vi "Append Numeric Table to Report.vi"(0 "report in":refnum<class "NI_Standard Report.lvclass">, 1 "column width (1)":dbl=1.0 format="%.2f", 2 "measurement system":u16(ring)=2 caption="measurement system for column width (Default)" items=["US", "Metric", "Default"], 3 "MS Office parameters":T2, 5 "column headers":string[](array[string]), 7 "row headers":string[](array[string]), 9 "numerical data":dbl[][](array[numeric]) format="%.2f", 11 "error in (no error)":errorcluster, 12 "format string (%.3f)":string="%.3f", 13 "separate page?":bool, 14 "show grid lines":bool=TRUE) -> (4 "report out":refnum<class "NI_Standard Report.lvclass">, 8 "range (wd) - start (xl)":T1, 10 "end (xl)":cluster{"row (xl) ":i32, "col (xl) ":i32}, 15 "error out":errorcluster)   [LabVIEW 2017, in "NI_Standard Report.lvclass"]
doc: "Appends a 2D array to a report as a table with the given column width. You can use this polymorphic VI to append an array of strings or numbers. The data type you wire to the <B>text data</B> input determines the polymorphic instance to use."
uses:
  <vilib>/Utility/NIReport.llb/Standard Report/NI_Standard Report.lvclass
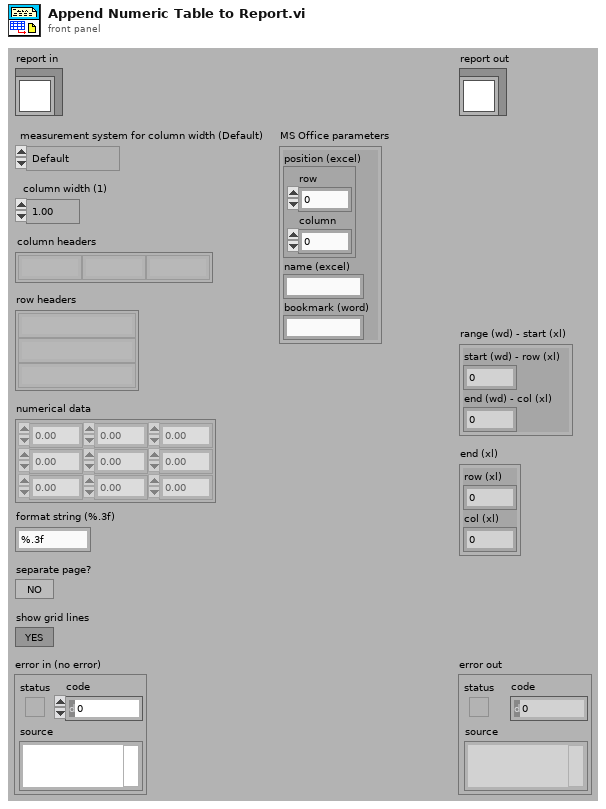
[diagram p1: front panel]
types:
  T1 = cluster{"start (wd) - row (xl) ":i32, "end (wd) - col (xl) ":i32}
  T2 = cluster{"position (excel)":cluster{"row":i32, "column":i32}, "name (excel)":string, "bookmark (word)":string}
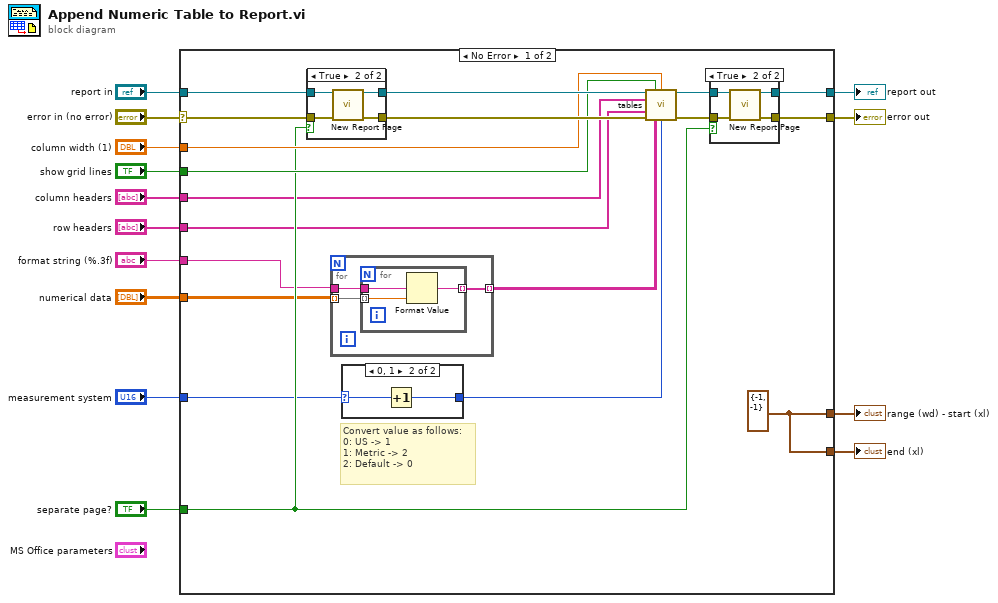
[diagram p0: block diagram]
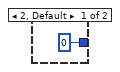
[diagram p2: hidden frame]
diagram:
  n1 = case shown="No Error" "error in (no error)" {
    selector: "error in (no error)" -> [w25 w56]
    tunnel: [w24 w56] -> w13
    tunnel: [w26 w55] -> w11
    tunnel: "report in" -> [w29 w55]
    tunnel: "show grid lines" -> [w22 _]
    tunnel: "format string (%.3f)" -> [w17 _]
    tunnel: "row headers" -> [w19 _]
    tunnel: "column headers" -> [w20 _]
    tunnel: "numerical data" -> [w18 _]
    tunnel: "column width (1)" -> [w23 _]
    tunnel: "separate page?" -> [w21 _]
    tunnel: "measurement system" -> [w16 _]
    tunnel: [w15 _] -> w2
    tunnel: [w15 _] -> w1
    frame No Error {
      w15 = cluster{"row (xl)":i32, "col (xl)":i32} {"row (xl)"=-1, "col (xl)"=-1} ("end (xl)")
      # "Convert value as follows:\n0: US -> 1\n1: Metric -> 2\n2: Default -> 0"
      n2 = case shown="True" w21 {
        tunnel: w29 -> [w50 w54]
        tunnel: w25 -> [w49 w53]
        tunnel: [w50 w52] -> w28
        tunnel: [w49 w51] -> w30
        frame False {
        }
        frame True {
          n3 = call-dynamic "New Report Page.vi"("report in"=w54, "error in (no error)"=w53) -> ("report out"=w52:refnum<class "NI_Standard Report.lvclass">, "error out"=w51:errorcluster)  [unwired: 1 in, 11 out]
        }
      }
      n4 = for {
        tunnel: w18 -> [w39] mode=indexing
        tunnel: w17 -> [w38]
        tunnel: [w37] -> w32 mode=indexing
        n5 = for {
          tunnel: w39 -> [w42] mode=indexing
          tunnel: w38 -> [w41]
          tunnel: [w40] -> w37 mode=indexing
          n6 = Format Value(format string=w41, value (0)=w42) -> (output string=w40:string)  [unwired: 1 out]
        }
      }
      n7 = case shown="0, 1" w16 {
        selector: w16 -> [_ w36]
        tunnel: [u16 0 w35] -> w33
        frame 2, Default {
        }
        frame 0, 1 {
          n8 = Increment(x=w36) -> (x+1=w35:u16)
        }
      }
      n9 = call <vilib>:"tables.vi"("report in"=w28, "show grid lines"=w22, "column width"=w23, "column headers"=w20, "row headers"=w19, "error in (no error)"=w30, "text data"=w32, "Measurement System"=w33) -> ("report out"=w27:refnum<class "NI_Standard Report.lvclass">, "error out"=w31:errorcluster)  [unwired: 6 out]
      n10 = case shown="True" w21 {
        tunnel: w27 -> [w44 w48]
        tunnel: w31 -> [w43 w47]
        tunnel: [w44 w46] -> w26
        tunnel: [w43 w45] -> w24
        frame False {
        }
        frame True {
          n11 = call-dynamic "New Report Page.vi"("report in"=w48, "error in (no error)"=w47) -> ("report out"=w46:refnum<class "NI_Standard Report.lvclass">, "error out"=w45:errorcluster)  [unwired: 1 in, 11 out]
        }
      }
    }
    frame Error {
    }
  }
  "error out" <- w13
  "report out" <- w11
  "end (xl)" <- w1
  "range (wd) - start (xl)" <- w2
